vi "flip_array.vi"(1 "input array":i32[][](array[numeric]), 2 "H/V":bool) -> (0 "OutputArray":i32[][](graph))   [LabVIEW 2009]
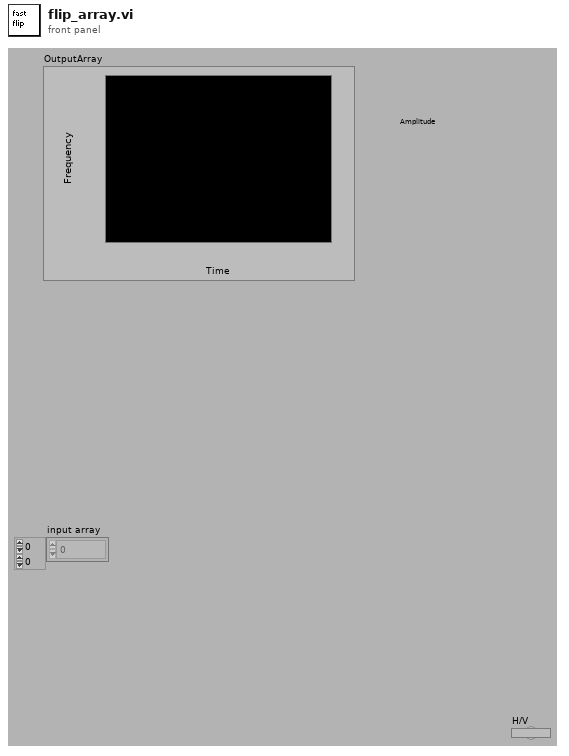
[diagram p1: front panel]
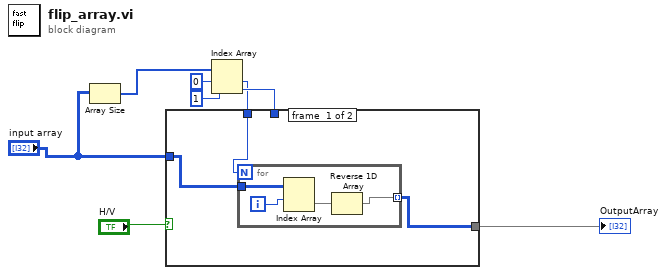
[diagram p0: block diagram]
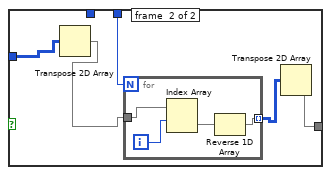
[diagram p2: hidden frame]
diagram:
  n1 = Array Size(array="input array") -> (size(s)=w5:i32[])
  n2 = Index Array(array=w5, index #1=0 ("index"), index #2=1 ("index")) -> (element #1=w1:i32, element #2=w2:i32)
  n3 = case shown="False" "H/V" {
    tunnel: "input array" -> [w11 w18]
    tunnel: [w10 w19] -> w7
    tunnel: w2 -> [_ w16]
    tunnel: w1 -> [w9 _]
    frame #0 {
      n4 = for {
        N: w9 -> [_]
        tunnel: w11 -> [w15]
        tunnel: [w13] -> w10 mode=indexing
        i -> [w12]
        n5 = Index Array(array=w15, index (row)=w12) -> (element=w14:i32[])  [unwired: 1 in]
        n6 = Reverse 1D Array(array=w14) -> (reversed array=w13:i32[])
      }
    }
    frame #1 {
      n7 = Transpose 2D Array(2D array=w18) -> (transposed array=w17:i32[][])
      n8 = for {
        N: w16 -> [_]
        tunnel: [w23] -> w20 mode=indexing
        tunnel: w17 -> [w22]
        i -> [w21]
        n9 = Index Array(array=w22, index (row)=w21) -> (element=w24:i32[])  [unwired: 1 in]
        n10 = Reverse 1D Array(array=w24) -> (reversed array=w23:i32[])
      }
      n11 = Transpose 2D Array(2D array=w20) -> (transposed array=w19:i32[][])
    }
  }
  "OutputArray" <- w7
